vi "Support Global.vi"() -> ()   [LabVIEW 2018]
uses:
  Wavelength Cluster Variable.ctl
panel:
  in  "Wavelength Variable":T1={"Filter Num"=1, "Grating Density"=0, "Wavelength(nm)"=0}
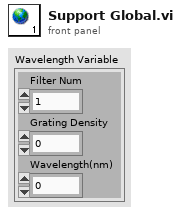
[diagram p1: front panel]
types:
  T1 = typedef "Wavelength Cluster Variable.ctl" = cluster{"Filter Num":i32, "Grating Density":i32, "Wavelength(nm)":i32}
diagram:
